vi "Phsae_shift_test(1).vi"() -> ()   [LabVIEW 2017]
uses:
  <vilib>/Analysis/3filter.llb/Filter Passband Type.ctl
  <vilib>/Analysis/4window.llb/windowTd.ctl
  <vilib>/measure/maspectr.llb/FFT Spectrum (Real-Im) for 1 Chan.vi
  <vilib>/Analysis/3filter.llb/FIR Windowed Filter (DBL).vi
  <vilib>/Analysis/NI_AALBase.lvlib
  <vilib>/Analysis/NI_AALPro.lvlib
  <vilib>/measure/NI_MAPro.lvlib
panel:
  out "S1 LPF out FFT(amplitude)":waveform(dbl)(graph)
  out "S1 LPF out FFT(Phase)":waveform(dbl)(graph)
  out "S0 LPF out FFT(amplitude)":waveform(dbl)(graph)
  out "S0 LPF out FFT(Phase)":waveform(dbl)(graph)
  out "S0 LPF output":waveform(dbl)(graph)
  out "S1 LPF output":waveform(dbl)(graph)
  out "S1 FFT(amplitude) 2":waveform(dbl)(graph)
  out "S1 FFT(Phase)":waveform(dbl)(graph)
  out "S0 FFT(amplitude)":waveform(dbl)(graph)
  out "S0 FFT(Phase)":waveform(dbl)(graph)
  out "S1 signal":waveform(dbl)(graph)
  in  "Message Signal Phsae":dbl
  in  "Carrier Frequency(Hz)":dbl
  in  "Frequency(Hz)":dbl
  in  "Amplitude(Vpeak)":dbl
  in  "Pulse length(sec)":dbl
  in  "Sampling frequency(Hz)":dbl
  in  "Delay time.A.1(sec)":dbl
  out "크기":i32
  out "S0 signal":waveform(dbl)(graph)
  out "Pulse SIG":dbl[](array[numeric])
  out "Delay SIG.A.1":dbl[](array[numeric])
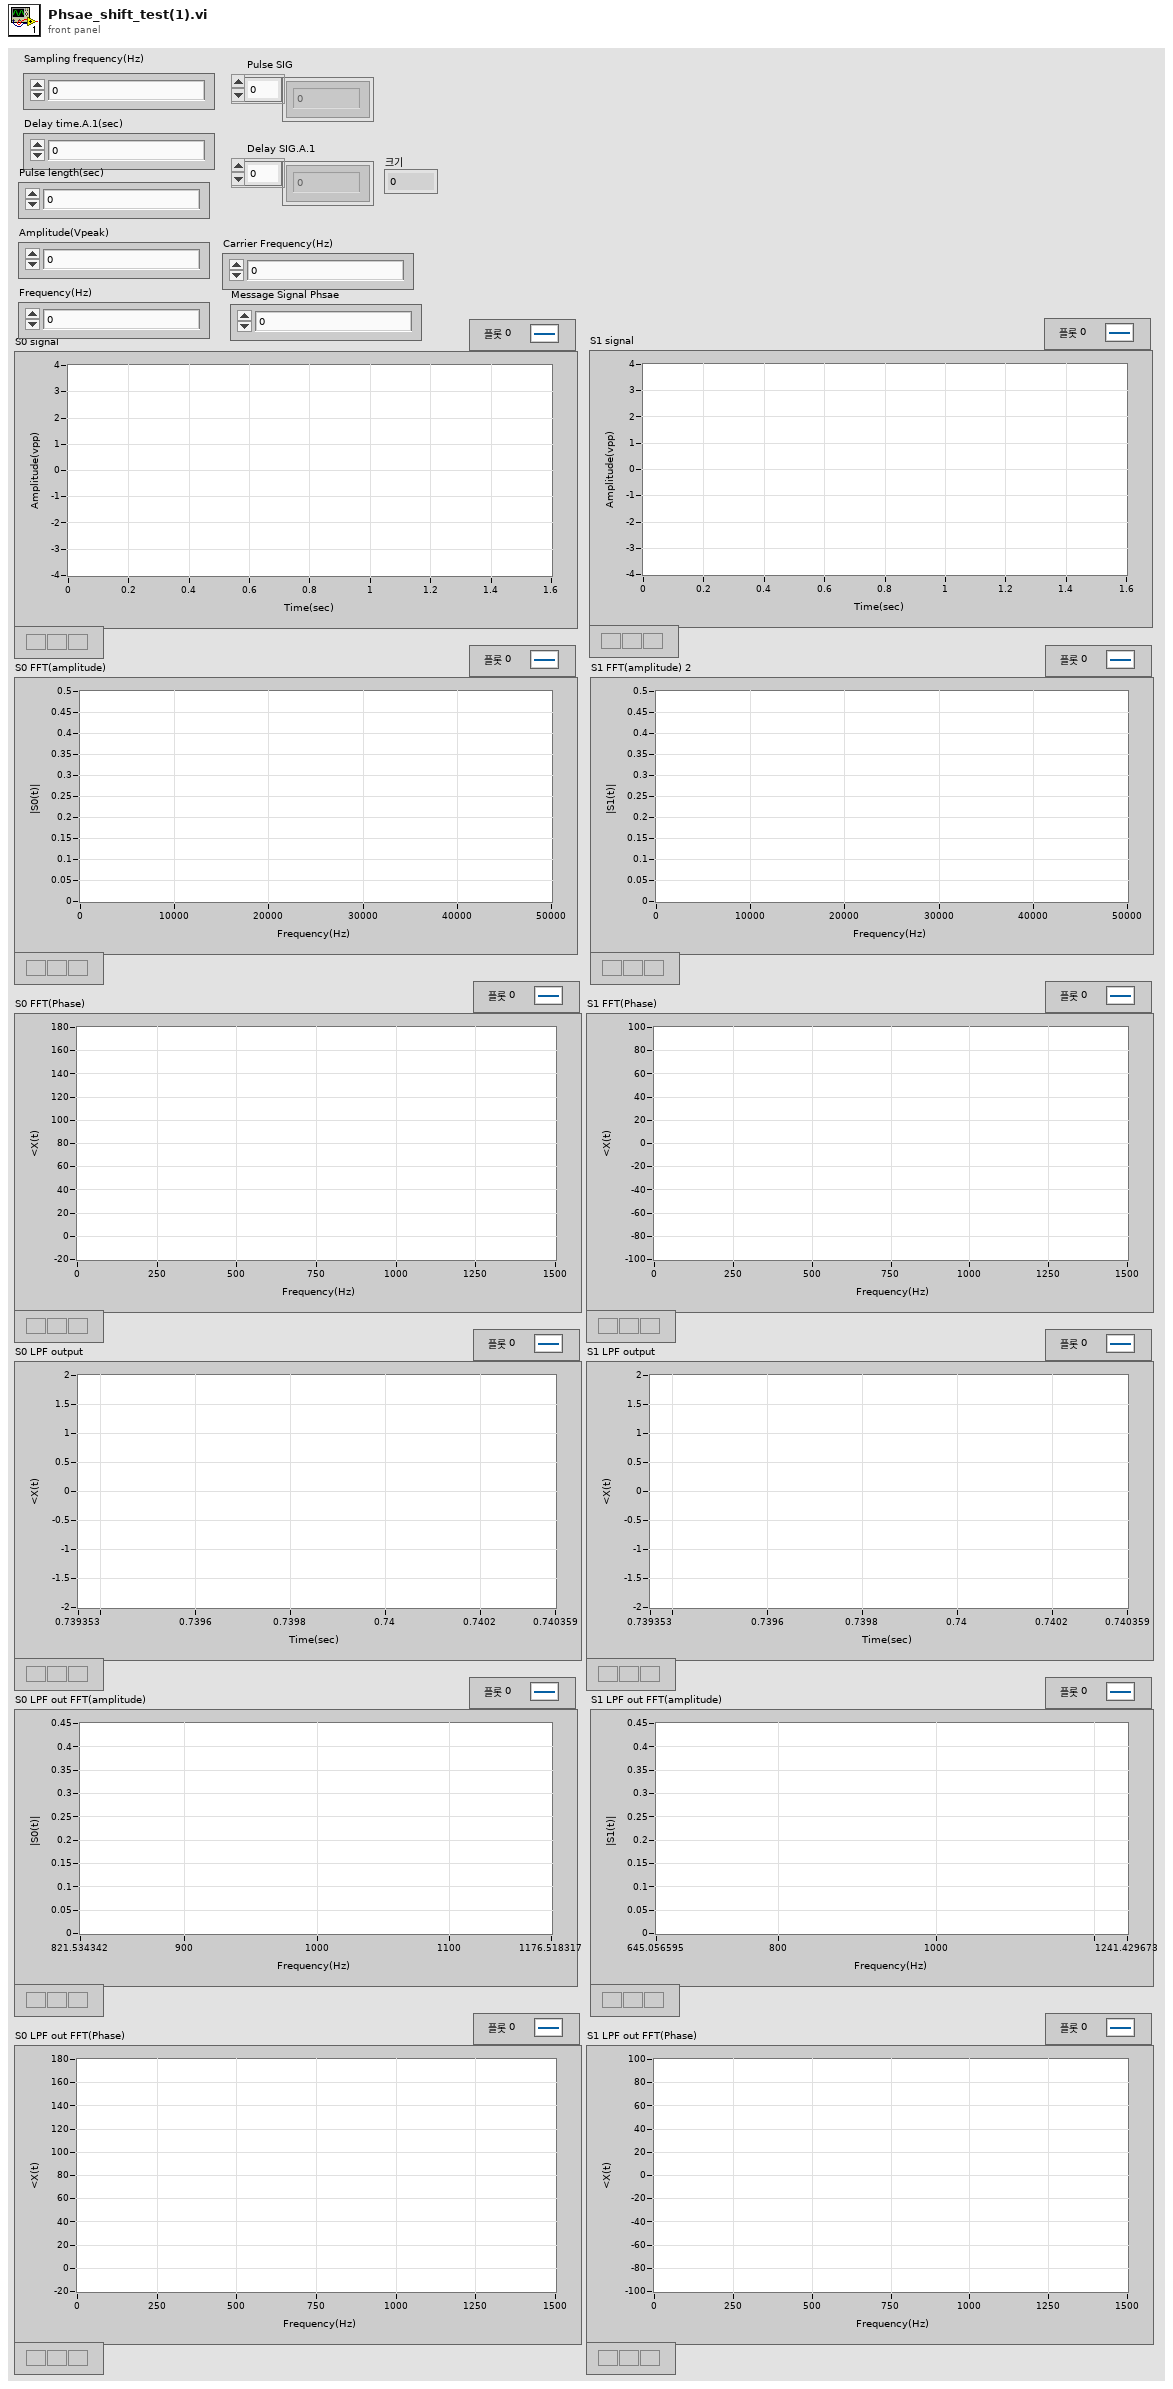
[diagram p1: front panel]
types:
  T1 = typedef "NI_AALBase.lvlib/Filter Passband Type.ctl" = enum32{"Lowpass", "Highpass", "Bandpass", "Bandstop"}
  T2 = cluster{"f0":dbl, "df":dbl, "imaginary part":dbl[]}
  T3 = typedef "NI_AALPro.lvlib/windowTd.ctl" = u32
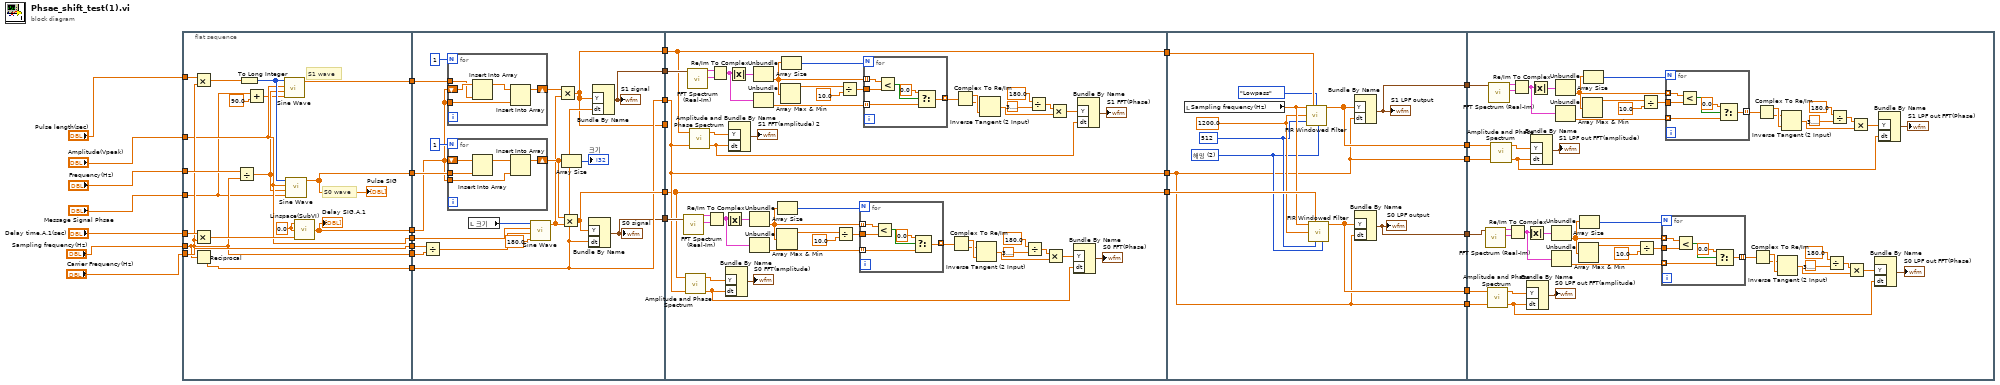
[diagram p0: block diagram]
diagram:
  n1 = flat-sequence {
    tunnel: "Frequency(Hz)" -> [w44]
    tunnel: "Amplitude(Vpeak)" -> [w35]
    tunnel: "Pulse length(sec)" -> [w43]
    tunnel: "Sampling frequency(Hz)" -> [w38]
    tunnel: "Delay time.A.1(sec)" -> [w42]
    tunnel: [w37] -> w29
    tunnel: [w41] -> w28
    tunnel: [w40] -> w27
    tunnel: [w35] -> w26
    tunnel: "Carrier Frequency(Hz)" -> [w39]
    tunnel: [w39] -> w25
    tunnel: [w38] -> w24
    tunnel: [w33] -> w17
    tunnel: "Message Signal Phsae" -> [w30]
    tunnel: w29 -> [w66]
    tunnel: w28 -> [w55]
    tunnel: w27 -> [w51]
    tunnel: w26 -> [w64]
    tunnel: w25 -> [w60]
    tunnel: w24 -> [w59]
    tunnel: w17 -> [w56]
    tunnel: [w50] -> w15
    tunnel: [w51] -> w14
    tunnel: [w52] -> w13
    tunnel: [w50] -> w12
    tunnel: [w49] -> w11
    tunnel: [w48] -> w10
    tunnel: w13 -> [w78]
    tunnel: w14 -> [w79]
    tunnel: w15 -> [w81]
    tunnel: w12 -> [_]
    tunnel: w11 -> [w111]
    tunnel: w10 -> [w83]
    tunnel: [w81] -> w9
    tunnel: [w79] -> w8
    tunnel: [w78] -> w7
    tunnel: w9 -> [w150]
    tunnel: w8 -> [w139]
    tunnel: w7 -> [w148]
    tunnel: [w143] -> w6
    tunnel: [w142] -> w5
    tunnel: [w139] -> w4
    tunnel: [w141] -> w3
    tunnel: [w140] -> w2
    tunnel: [w139] -> w1
    tunnel: w6 -> [w156]
    tunnel: w5 -> [w155]
    tunnel: w4 -> [w154]
    tunnel: w3 -> [w153]
    tunnel: w2 -> [w152]
    tunnel: w1 -> [w151]
    frame #0 {
      w45 = 0.0 ("frequency")
      # "S1 wave"
      # "S0 wave"
      n2 = Multiply(x=w43, y=w38) -> (x*y=w47:dbl)
      n3 = Multiply(x=w42, y=w38) -> (x*y=w46:dbl)
      n4 = Reciprocal(x=w38) -> (1/x=w40:dbl)
      n5 = Divide(x=w44, y=w38) -> (x/y=w34:dbl)
      n6 = To Long Integer(number=w47) -> (32bit integer=w36:i32)
      n7 = Add(x=w30, y=90.0) -> (x+y=w31:dbl)
      n8 = call <vilib>:"Sine Wave.vi"("samples"=w36, "amplitude"=w35, "frequency"=w34, "phase in"=w31) -> ("sine wave"=w33:dbl[])  [unwired: 1 in, 2 out]
      n9 = call <vilib>:"Sine Wave.vi"("samples"=w36, "amplitude"=w35, "frequency"=w34, "phase in"=w30) -> ("sine wave"=w37:dbl[])  [unwired: 1 in, 2 out]
      "Pulse SIG" <- w37
      n10 = call "Linspace(SubVI).vi"("NumElements"=w46, "End"=w45, "Start"=w45) -> ("Array"=w41:dbl[])
      "Delay SIG.A.1" <- w41
    }
    frame #1 {
      n11 = Divide(x=w60, y=w59) -> (x/y=w61:dbl)
      n12 = for {
        N: 1 -> [_]
        shift-right: [w68] -> w54
        shift-left: w55 -> [w72]
        tunnel: w56 -> [w71]
        tunnel: w55 -> [w69]
        n13 = Insert Into Array(array=w72, new element=w71) -> (w70:dbl[])  [unwired: 1 in]
        n14 = Insert Into Array(array=w70, new element=w69) -> (w68:dbl[])  [unwired: 1 in]
      }
      n15 = for {
        N: 1 -> [_]
        shift-right: [w73] -> w58
        shift-left: w55 -> [w77]
        tunnel: w66 -> [w76]
        tunnel: w55 -> [w74]
        n16 = Insert Into Array(array=w77, new element=w76) -> (w75:dbl[])  [unwired: 1 in]
        n17 = Insert Into Array(array=w75, new element=w74) -> (w73:dbl[])  [unwired: 1 in]
      }
      n18 = local read "크기"() -> (w62:i32)
      n19 = call <vilib>:"Sine Wave.vi"("samples"=w62, "amplitude"=w64, "frequency"=w61, "phase in"=180.0) -> ("sine wave"=w53:dbl[])  [unwired: 1 in, 2 out]
      n20 = Multiply(x=w54, y=w53) -> (x*y=w50:dbl[])
      n21 = Multiply(x=w58, y=w53) -> (x*y=w52:dbl[])
      n22 = Array Size(array=w58) -> (size(s)=→"크기":i32)
      n23 = Bundle By Name("Y"=w52, "dt"=w51) -> (w49:waveform(dbl))  [unwired: 1 in]
      "S0 signal" <- w49
      n24 = Bundle By Name("Y"=w50, "dt"=w51) -> (w48:waveform(dbl))  [unwired: 1 in]
      "S1 signal" <- w48
    }
    frame #2 {
      n25 = call-poly <vilib>:"FFT Spectrum (Real-Im).vi"("time signal"=w111) -> ("imaginary part"=w109:T2, "real part"=w110:cluster{"f0":dbl, "df":dbl, "real part":dbl[]})  [unwired: 6 in, 3 out]
      n26 = call <vilib>:"Amplitude and Phase Spectrum.vi"("dt"=w79, "Signal (V)"=w78) -> ("df"=w105:dbl, "Amp Spectrum Mag (Vrms)"=w107:dbl[])  [unwired: 1 in, 1 out]
      n27 = call-poly <vilib>:"FFT Spectrum (Real-Im).vi"("time signal"=w83) -> ("imaginary part"=w87:T2, "real part"=w88:cluster{"f0":dbl, "df":dbl, "real part":dbl[]})  [unwired: 6 in, 3 out]
      n28 = call <vilib>:"Amplitude and Phase Spectrum.vi"("dt"=w79, "Signal (V)"=w81) -> ("df"=w80:dbl, "Amp Spectrum Mag (Vrms)"=w85:dbl[])  [unwired: 1 in, 1 out]
      n29 = Re/Im To Complex(1:w109, 2:w110) -> (0:w108:cluster{"f0":cdb, "df":cdb, cdb[]})
      n30 = Re/Im To Complex(1:w87, 2:w88) -> (0:w86:cluster{"f0":cdb, "df":cdb, cdb[]})
      n31 = Absolute Value(x=w108) -> (abs(x)=w126:cluster{"f0":dbl, "df":dbl, dbl[]})
      n32 = Bundle By Name("Y"=w107, "dt"=w105) -> (→"S0 FFT(amplitude)":waveform(dbl))  [unwired: 1 in]
      n33 = Absolute Value(x=w86) -> (abs(x)=w104:cluster{"f0":dbl, "df":dbl, dbl[]})
      n34 = Bundle By Name("Y"=w85, "dt"=w80) -> (→"S1 FFT(amplitude) 2":waveform(dbl))  [unwired: 1 in]
      n35 = Unbundle(w126) -> (w115:dbl[])  [unwired: 2 out]
      n36 = Unbundle(w108) -> (w112:cdb[])  [unwired: 2 out]
      n37 = Unbundle(w104) -> (w92:dbl[])  [unwired: 2 out]
      n38 = Unbundle(w86) -> (w89:cdb[])  [unwired: 2 out]
      n39 = Array Max & Min(array=w115) -> (max value=w114:dbl)  [unwired: 3 out]
      n40 = Array Size(array=w115) -> (size(s)=w116:i32)
      n41 = Array Max & Min(array=w92) -> (max value=w91:dbl)  [unwired: 3 out]
      n42 = Array Size(array=w92) -> (size(s)=w93:i32)
      n43 = Divide(x=w114, y=10.0) -> (x/y=w125:dbl)
      n44 = Divide(x=w91, y=10.0) -> (x/y=w103:dbl)
      n45 = for {
        N: w116 -> [_]
        tunnel: [w136] -> w117 mode=indexing
        tunnel: w115 -> [w135] mode=indexing
        tunnel: w125 -> [w134]
        tunnel: w112 -> [w133] mode=indexing
        n46 = Less?(x=w135, y=w134) -> (x < y?=w138:bool)
        n47 = Select(t=0.0, s=w138, f=w133) -> (s? t:f=w136:cdb)
      }
      n48 = for {
        N: w93 -> [_]
        tunnel: [w130] -> w94 mode=indexing
        tunnel: w92 -> [w129] mode=indexing
        tunnel: w103 -> [w128]
        tunnel: w89 -> [w127] mode=indexing
        n49 = Less?(x=w129, y=w128) -> (x < y?=w132:bool)
        n50 = Select(t=0.0, s=w132, f=w127) -> (s? t:f=w130:cdb)
      }
      n51 = Complex To Re/Im(x + iy=w117) -> (x=w124:dbl[], y=w123:dbl[])
      n52 = Complex To Re/Im(x + iy=w94) -> (x=w102:dbl[], y=w101:dbl[])
      n53 = Inverse Tangent (2 Input)(1:w124, 2:w123) -> (0:w120:dbl[])
      n54 = Inverse Tangent (2 Input)(1:w102, 2:w101) -> (0:w97:dbl[])
      n55 = Divide(x=180.0, y=3.141592653589793) -> (x/y=w119:dbl)
      n56 = Divide(x=180.0, y=3.141592653589793) -> (x/y=w96:dbl)
      n57 = Multiply(x=w119, y=w120) -> (x*y=w118:dbl[])
      n58 = Multiply(x=w96, y=w97) -> (x*y=w95:dbl[])
      n59 = Bundle By Name("Y"=w118, "dt"=w105) -> (→"S0 FFT(Phase)":waveform(dbl))  [unwired: 1 in]
      n60 = Bundle By Name("Y"=w95, "dt"=w80) -> (→"S1 FFT(Phase)":waveform(dbl))  [unwired: 1 in]
    }
    frame #3 {
      w144 = T3 2 items=["사각형"=0, "해닝"=1, "해밍"=2, "블랙맨-해리스"=3, "정밀한 블랙맨"=4, "블랙맨"=5, "플랫 탑"=6, "4항 블랙맨-해리스 "=7, "7항 블랙맨-해리스"=8, "낮은 사이드로브"=9, "블랙맨 누탈"=11, "삼각형"=30, "바틀렛-해닝"=31, "보먼"=32, "파젠"=33, "웰치"=34, "카이저"=60, "돌프-체비셰프"=61, "가우스"=62] ("window")
      w145 = 512 ("taps")
      w146 = 1200.0 ("low cutoff freq: fl")
      n61 = local read "Sampling frequency(Hz)"() -> (w147:dbl)
      n62 = call-poly <vilib>:"FIR Windowed Filter.vi"("sampling freq: fs"=w147, "X"=w150, "filter type"=Filter_Passband_Type."Lowpass", "low cutoff freq: fl"=w146, "taps"=w145, "window"=w144) -> ("Filtered X"=w142:dbl[])  [unwired: 8 in, 1 out]
      n63 = call-poly <vilib>:"FIR Windowed Filter.vi"("sampling freq: fs"=w147, "X"=w148, "low cutoff freq: fl"=w146, "taps"=w145, "window"=w144) -> ("Filtered X"=w140:dbl[])  [unwired: 9 in, 1 out]
      n64 = Bundle By Name("Y"=w142, "dt"=w139) -> (w143:waveform(dbl))  [unwired: 1 in]
      "S1 LPF output" <- w143
      n65 = Bundle By Name("Y"=w140, "dt"=w139) -> (w141:waveform(dbl))  [unwired: 1 in]
      "S0 LPF output" <- w141
    }
    frame #4 {
      n66 = call-poly <vilib>:"FFT Spectrum (Real-Im).vi"("time signal"=w153) -> ("imaginary part"=w184:T2, "real part"=w185:cluster{"f0":dbl, "df":dbl, "real part":dbl[]})  [unwired: 6 in, 3 out]
      n67 = call <vilib>:"Amplitude and Phase Spectrum.vi"("dt"=w151, "Signal (V)"=w152) -> ("df"=w180:dbl, "Amp Spectrum Mag (Vrms)"=w182:dbl[])  [unwired: 1 in, 1 out]
      n68 = call-poly <vilib>:"FFT Spectrum (Real-Im).vi"("time signal"=w156) -> ("imaginary part"=w162:T2, "real part"=w163:cluster{"f0":dbl, "df":dbl, "real part":dbl[]})  [unwired: 6 in, 3 out]
      n69 = call <vilib>:"Amplitude and Phase Spectrum.vi"("dt"=w154, "Signal (V)"=w155) -> ("df"=w157:dbl, "Amp Spectrum Mag (Vrms)"=w160:dbl[])  [unwired: 1 in, 1 out]
      n70 = Re/Im To Complex(1:w184, 2:w185) -> (0:w183:cluster{"f0":cdb, "df":cdb, cdb[]})
      n71 = Re/Im To Complex(1:w162, 2:w163) -> (0:w161:cluster{"f0":cdb, "df":cdb, cdb[]})
      n72 = Absolute Value(x=w183) -> (abs(x)=w200:cluster{"f0":dbl, "df":dbl, dbl[]})
      n73 = Bundle By Name("Y"=w182, "dt"=w180) -> (→"S0 LPF out FFT(amplitude)":waveform(dbl))  [unwired: 1 in]
      n74 = Absolute Value(x=w161) -> (abs(x)=w179:cluster{"f0":dbl, "df":dbl, dbl[]})
      n75 = Bundle By Name("Y"=w160, "dt"=w157) -> (→"S1 LPF out FFT(amplitude)":waveform(dbl))  [unwired: 1 in]
      n76 = Unbundle(w200) -> (w189:dbl[])  [unwired: 2 out]
      n77 = Unbundle(w183) -> (w186:cdb[])  [unwired: 2 out]
      n78 = Unbundle(w179) -> (w167:dbl[])  [unwired: 2 out]
      n79 = Unbundle(w161) -> (w164:cdb[])  [unwired: 2 out]
      n80 = Array Max & Min(array=w189) -> (max value=w188:dbl)  [unwired: 3 out]
      n81 = Array Size(array=w189) -> (size(s)=w190:i32)
      n82 = Array Max & Min(array=w167) -> (max value=w166:dbl)  [unwired: 3 out]
      n83 = Array Size(array=w167) -> (size(s)=w168:i32)
      n84 = Divide(x=w188, y=10.0) -> (x/y=w199:dbl)
      n85 = Divide(x=w166, y=10.0) -> (x/y=w178:dbl)
      n86 = for {
        N: w190 -> [_]
        tunnel: [w210] -> w191 mode=indexing
        tunnel: w189 -> [w209] mode=indexing
        tunnel: w199 -> [w208]
        tunnel: w186 -> [w207] mode=indexing
        n87 = Less?(x=w209, y=w208) -> (x < y?=w212:bool)
        n88 = Select(t=0.0, s=w212, f=w207) -> (s? t:f=w210:cdb)
      }
      n89 = for {
        N: w168 -> [_]
        tunnel: [w204] -> w169 mode=indexing
        tunnel: w167 -> [w203] mode=indexing
        tunnel: w178 -> [w202]
        tunnel: w164 -> [w201] mode=indexing
        n90 = Less?(x=w203, y=w202) -> (x < y?=w206:bool)
        n91 = Select(t=0.0, s=w206, f=w201) -> (s? t:f=w204:cdb)
      }
      n92 = Complex To Re/Im(x + iy=w191) -> (x=w198:dbl[], y=w197:dbl[])
      n93 = Complex To Re/Im(x + iy=w169) -> (x=w177:dbl[], y=w176:dbl[])
      n94 = Inverse Tangent (2 Input)(1:w198, 2:w197) -> (0:w194:dbl[])
      n95 = Inverse Tangent (2 Input)(1:w177, 2:w176) -> (0:w172:dbl[])
      n96 = Divide(x=180.0, y=3.141592653589793) -> (x/y=w193:dbl)
      n97 = Divide(x=180.0, y=3.141592653589793) -> (x/y=w171:dbl)
      n98 = Multiply(x=w193, y=w194) -> (x*y=w192:dbl[])
      n99 = Multiply(x=w171, y=w172) -> (x*y=w170:dbl[])
      n100 = Bundle By Name("Y"=w192, "dt"=w180) -> (→"S0 LPF out FFT(Phase)":waveform(dbl))  [unwired: 1 in]
      n101 = Bundle By Name("Y"=w170, "dt"=w157) -> (→"S1 LPF out FFT(Phase)":waveform(dbl))  [unwired: 1 in]
    }
  }
